vi "oa_TV Average methods (NChan).vi"(5 "Window size":i16=10, 6 "channel index":i32, 7 "Enum":T1(ring)=enum."Moving average", 8 "previous date":cluster{dbl[][]}[](array[cluster]), 9 "Revulotion index":i32, 10 "Angle intervals":dbl[](array[numeric]), 11 "Array":dbl[][](array[numeric])) -> (0 "Previous data":cluster{dbl[][]}, 3 "Angle intervals":dbl[](array[numeric]))   [LabVIEW 2017, in "SoundVib_Torsional.lvlib"]
uses:
  <vilib>/addons/Sound and Vibration/Order Analysis/Torsional Vibration/SoundVib_Torsional.lvlib
  <vilib>/Analysis/baseanly.llb/Mean (DBL).vi
  <vilib>/Analysis/NI_AALBase.lvlib
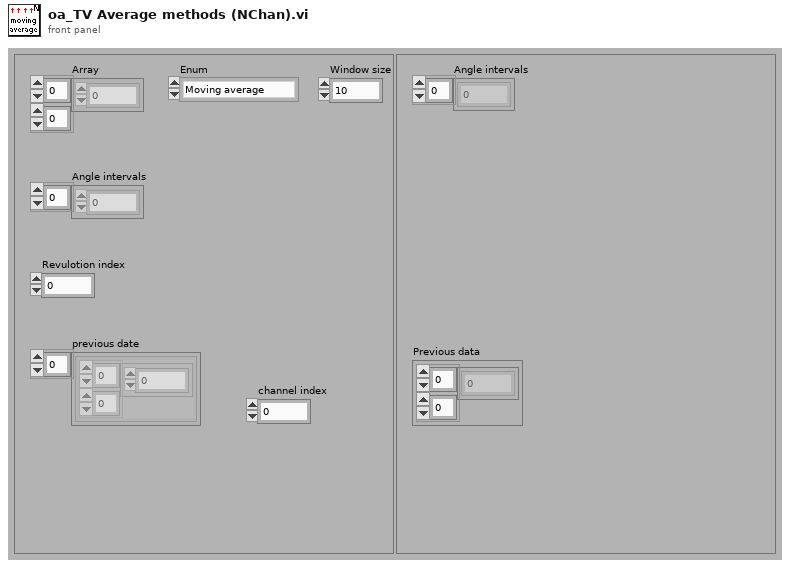
[diagram p1: front panel]
types:
  T1 = enum16{"Exponential average", "Moving average", "Current"}
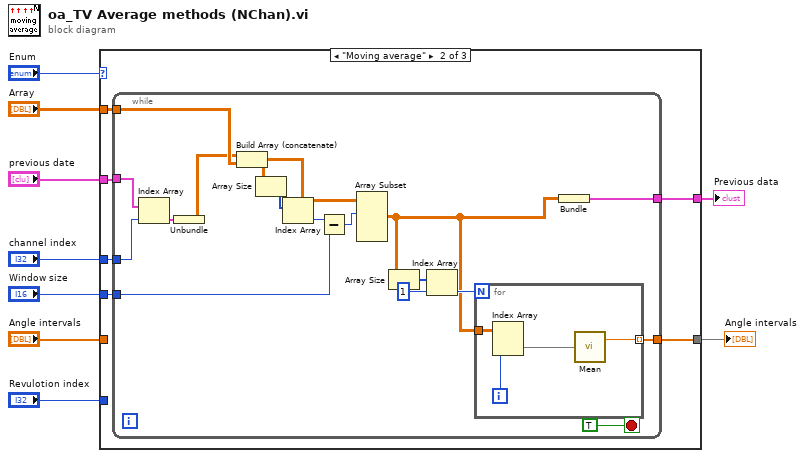
[diagram p0: block diagram]
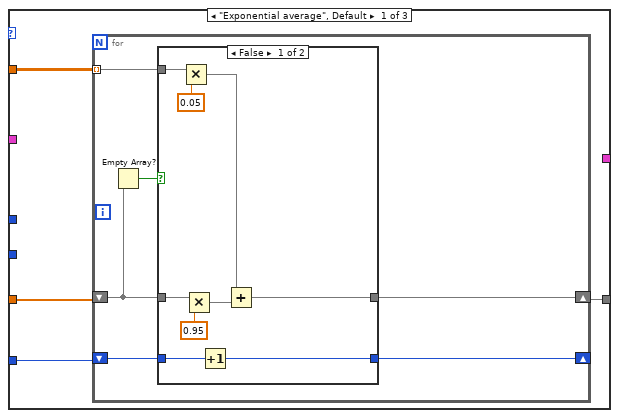
[diagram p2: hidden frame]
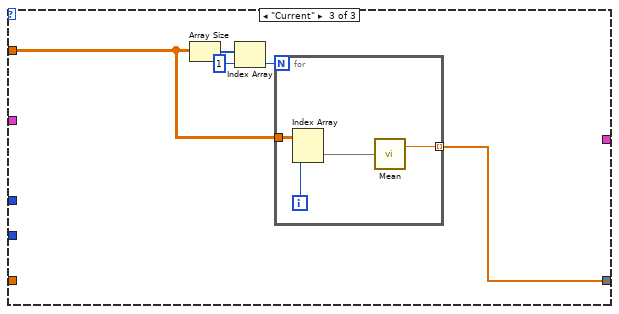
[diagram p4: hidden frame]
diagram:
  n1 = case shown="\"Moving average\"" "Enum" {
    tunnel: "Array" -> [w13 w36 w59]
    tunnel: "Angle intervals" -> [w12 _ _]
    tunnel: [w11 w34 w58] -> w7
    tunnel: "Revulotion index" -> [w10 _ _]
    tunnel: "Window size" -> [_ w35 _]
    tunnel: "channel index" -> [_ w33 _]
    tunnel: "previous date" -> [_ w32 _]
    tunnel: [_ w31 _] -> w1
    frame "Exponential average", Default {
      n2 = for {
        tunnel: w13 -> [w15] mode=indexing
        shift-right: [w18] -> _
        shift-left: w10 -> [w19]
        shift-right: [w14] -> w11
        shift-left: w12 -> [w17]
        n3 = Empty Array?(array=w17) -> (empty?=w16:bool)
        n4 = case shown="False" w16 {
          tunnel: [w20 w30] -> w14
          tunnel: w17 -> [w28 _]
          tunnel: w19 -> [w27 w29]
          tunnel: [w26 w29] -> w18
          tunnel: w15 -> [w23 w30]
          frame False {
            n5 = Multiply(x=w23, y=0.05 ("x+1")) -> (x*y=w21:dbl[])
            n6 = Multiply(x=w28, y=0.95 ("x+1")) -> (x*y=w25:dbl[])
            n7 = Increment(x=w27) -> (x+1=w26:i32)
            n8 = Add(x=w21, y=w25) -> (x+y=w20:dbl[])
          }
          frame True {
          }
        }
      }
    }
    frame "Moving average" {
      n9 = while {
        tunnel: w36 -> [w53]
        tunnel: w35 -> [w48]
        tunnel: [w43] -> w34
        tunnel: w33 -> [w38]
        tunnel: w32 -> [w41]
        tunnel: [w37] -> w31
        stop <- TRUE stop-if-true
        n10 = Index Array(array=w41, index=w38) -> (element=w40:cluster{dbl[][]})
        n11 = Unbundle(w40) -> (w39:dbl[][])
        n12 = Build Array (concatenate)(w39, w53) -> (w51:dbl[][])
        n13 = Array Size(array=w51) -> (size(s)=w50:i32[])
        n14 = Index Array(array=w50) -> (element=w49:i32)  [unwired: 1 in]
        n15 = Subtract(x=w49, y=w48) -> (x-y=w47:i32)
        n16 = Array Subset(array=w51, index (row)=w47) -> (w42:dbl[][])  [unwired: 3 in]
        n17 = Array Size(array=w42) -> (size(s)=w46:i32[])
        n18 = Index Array(array=w46, index=1) -> (element=w44:i32)
        n19 = for {
          N: w44 -> [_]
          tunnel: w42 -> [w57]
          tunnel: [w54] -> w43 mode=indexing
          i -> [w56]
          n20 = Index Array(array=w57, index (col)=w56) -> (element=w55:dbl[])  [unwired: 1 in]
          n21 = call-poly <vilib>:"Mean.vi"("X"=w55) -> ("mean"=w54:dbl)  [unwired: 1 out]
        }
        n22 = Bundle(w42) -> (w37:cluster{dbl[][]})  [unwired: 1 in]
      }
    }
    frame "Current" {
      n23 = Array Size(array=w59) -> (size(s)=w62:i32[])
      n24 = Index Array(array=w62, index=1) -> (element=w60:i32)
      n25 = for {
        N: w60 -> [_]
        tunnel: w59 -> [w66]
        tunnel: [w63] -> w58 mode=indexing
        i -> [w65]
        n26 = Index Array(array=w66, index (col)=w65) -> (element=w64:dbl[])  [unwired: 1 in]
        n27 = call-poly <vilib>:"Mean.vi"("X"=w64) -> ("mean"=w63:dbl)  [unwired: 1 out]
      }
    }
  }
  "Angle intervals" <- w7
  "Previous data" <- w1
